vi "Dark Current Test with Manual Measurment.vi"() -> ()   [LabVIEW 2018]
uses:
  <vilib>/Utility/file.llb/Write Delimited Spreadsheet (string).vi
  <vilib>/Utility/file.llb/Write Delimited Spreadsheet (DBL).vi
  <instrlib>/CAEN PSM/CAEN PSM.lvlib
panel:
  out "Power Supply Trip":bool
  out "Time Left (s)":dbl
  out "8":bool
  out "7":bool
  out "6":bool
  out "5":bool
  out "4":bool
  out "3":bool
  out "2":bool
  out "1":bool
  out "Test is Running":bool
  in  "Begin Test":bool
  out "Manual Measurments \nNeeded":bool
  out "OVV? 2":bool=TRUE
  out "OVC? 2":bool=TRUE
  out "Actual Voltage Level (V) 2":dbl format="%#_13g"
  out "Recorded Current\nfor Previous Tube":dbl format="%#_13g"
  in  "Measure Next Tube":bool
  in  "Barcodes":string[](array[string])
  out "Next Measurment":string
  in  "N":i32
  in  "dt (s)":i32
  out "Actual Current Limit (nA)":dbl format="%#_13g"
  out "Actual Voltage Level (V)":dbl format="%#_13g"
  out "OVC?":bool=TRUE
  out "OVV?":bool=TRUE
  in  "Channel #":i32
  in  "VISA resource name":refnum<visa-resource-name>
  # "Dark Current Test"
  # "Instructions in Brief:\n1. Begin the program by clicking the white arrow.\n2. Assemble tubes into the test bench.\n3. Select COM5 for the \"VISA resource name\".\n4. Enter in how often you want to take measurement in the \"dt\" box (typically 60s)\n5. Enter in how many measurments you want to take (typically 15)\n6. Scan in the 8 tubes that you are testing.\n(If you take 15 measurments every 60s, the test will take 15 min.)\n7. Click \"Begin Test\". The \"Test is Running\" LED should light up.\n8. After the intial test, if the total current is below 16nA, \n    the program will write the \n     file and end the test.\n9. If the total current is above 16nA, manual\n    measurments need to be taken.\n10. Engage only the tube indicated by \"Next Measurment\". \n11. Click \"Measure\".\n12. Engage the next tube and continue untill all have been measured.\n13. In both cases, the program will write files and end the test. \n14. The test is over when the \"Test is Running\" LED has turned off."
  # "Green lights indicate tubes that have passed."
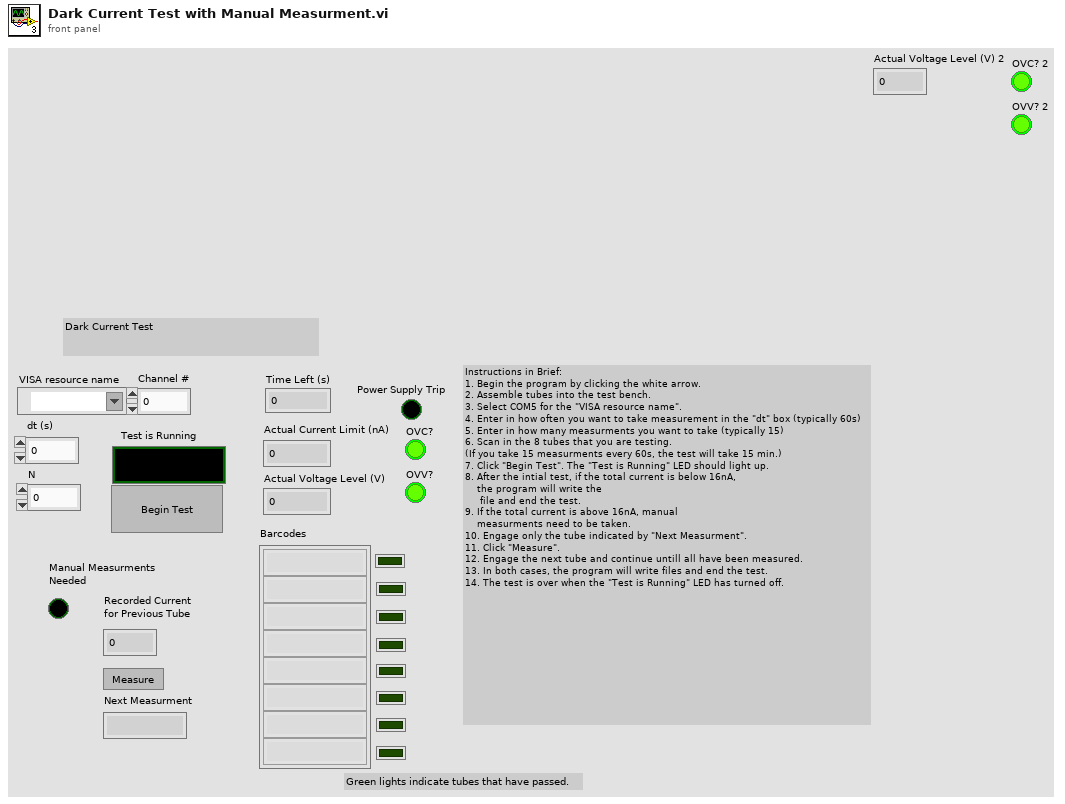
[diagram p1: front panel]
types:
  T1 = typedef "CAEN PSM.lvlib/BoardHandle.ctl" = cluster{"VISA resource name":refnum<visa-resource-name>, "Board address":u8, "NChannels":u8}
  T2 = cluster{"ON":bool, "RUP":bool, "RDW":bool, "OVC":bool, "OVV":bool, "UNV":bool, "MAXV":bool, "TRIP":bool, "OVP":bool, "OVT":bool, "DIS":bool, "KILL":bool, "ILK":bool, "NOCAL":bool}[]
  T3 = cluster{"ON":bool, "RUP":bool, "RDW":bool, "OVC":bool, "OVV":bool, "UNV":bool, "MAXV":bool, "TRIP":bool, "OVP":bool, "OVT":bool, "DIS":bool, "KILL":bool, "ILK":bool, "NOCAL":bool}
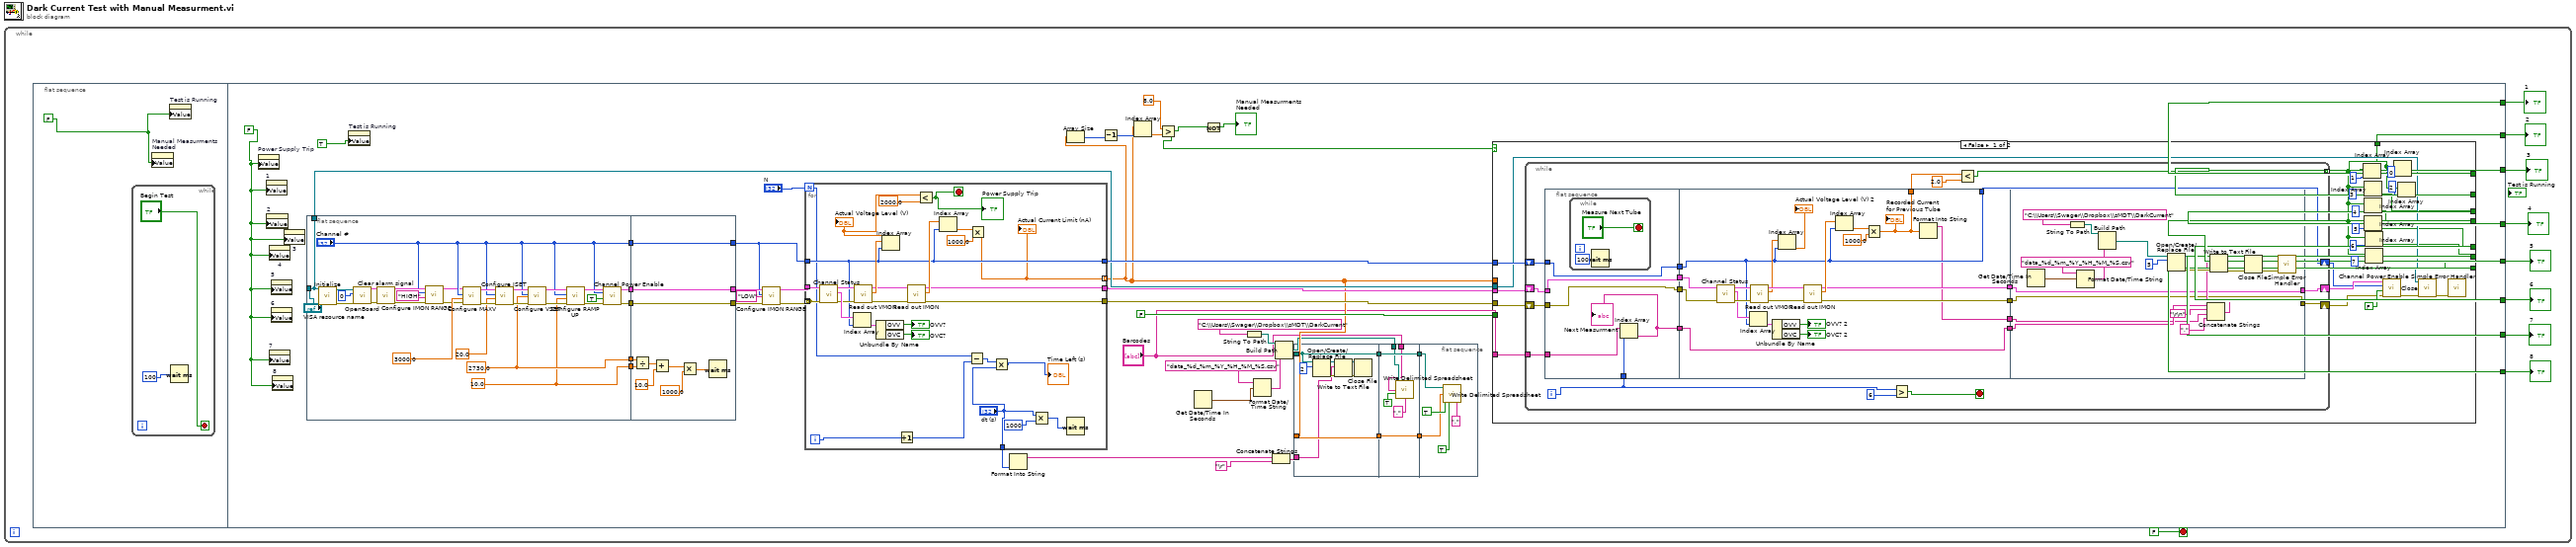
[diagram p0: block diagram]
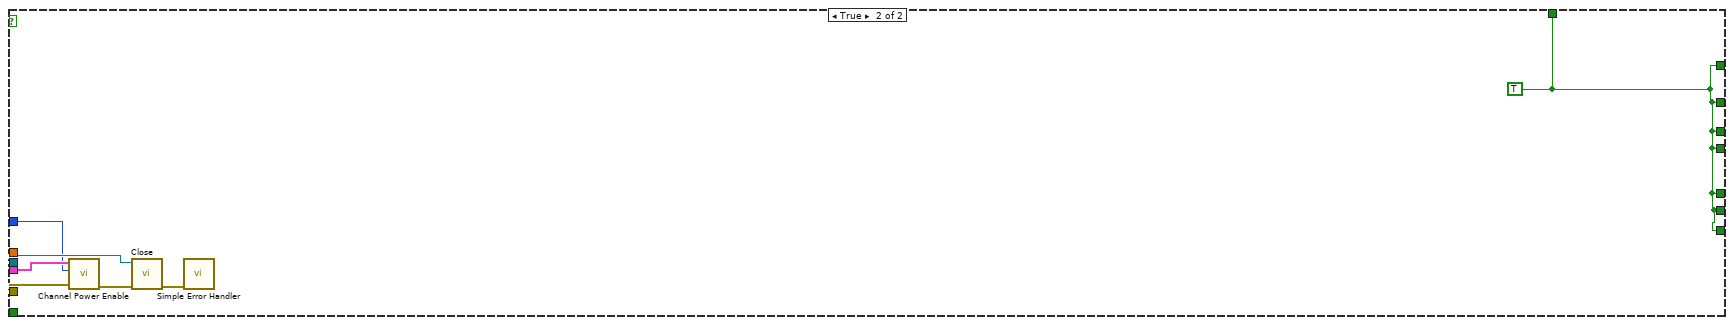
[diagram p2: hidden frame]
diagram:
  n1 = while {
    stop <- FALSE stop-if-true
    n2 = flat-sequence {
      tunnel: [w37] -> w8
      tunnel: [w36] -> w7
      tunnel: [w35] -> w6
      tunnel: [w34] -> w5
      tunnel: [w33] -> w4
      tunnel: [w32] -> w3
      tunnel: [w31] -> w2
      tunnel: [w30] -> w1
      frame #0 {
        w10 = FALSE
        n3 = while {
          stop <- "Begin Test" stop-if-true
          n4 = Wait (ms)(milliseconds to wait=100) -> ()  [unwired: 1 out]
        }
        n5 = property on="Manual Measurments \nNeeded" class="Bool (strict)"("Value"=w10) -> ()  [unwired: 2 in, 2 out]
        n6 = property on="Test is Running" class="Bool (strict)"("Value"=w10) -> ()  [unwired: 2 in, 2 out]
      }
      frame #1 {
        w23 = FALSE
        n7 = property on="Power Supply Trip" class="Bool (strict)"("Value"=w23) -> ()  [unwired: 2 in, 2 out]
        n8 = property on="1" class="Bool (strict)"("Value"=w23) -> ()  [unwired: 2 in, 2 out]
        n9 = property on="2" class="Bool (strict)"("Value"=w23) -> ()  [unwired: 2 in, 2 out]
        n10 = property on="4" class="Bool (strict)"("Value"=w23) -> ()  [unwired: 2 in, 2 out]
        n11 = property on="7" class="Bool (strict)"("Value"=w23) -> ()  [unwired: 2 in, 2 out]
        n12 = property on="5" class="Bool (strict)"("Value"=w23) -> ()  [unwired: 2 in, 2 out]
        n13 = property on="6" class="Bool (strict)"("Value"=w23) -> ()  [unwired: 2 in, 2 out]
        n14 = property on="8" class="Bool (strict)"("Value"=w23) -> ()  [unwired: 2 in, 2 out]
        n15 = property on="3" class="Bool (strict)"("Value"=w23) -> ()  [unwired: 2 in, 2 out]
        n16 = flat-sequence {
          tunnel: [w197] -> w62
          tunnel: [w196] -> w61
          tunnel: [w193] -> w52
          tunnel: [w195] -> w60
          tunnel: [w194] -> w59
          tunnel: ["Channel #"] -> w58
          tunnel: "VISA resource name" -> [w193]
          tunnel: w62 -> [w217]
          tunnel: w61 -> [w216]
          tunnel: [w215] -> w49
          tunnel: w60 -> [w215]
          tunnel: [w214] -> w50
          tunnel: w59 -> [w214]
          tunnel: [w213] -> w47
          tunnel: w58 -> [w213]
          frame #0 {
            w197 = 2730.0 ("Voltage Set (Volts)")
            w196 = 10.0 ("Voltage Ramp Up (V/s)")
            n17 = call <instrlib>:"Initialize.vi"("VISA resource name"=w193) -> ("error out"=w207:errorcluster, "VISA resource name out"=w203:refnum<visa-resource-name>)  [unwired: 9 in]
            n18 = call <instrlib>:"OpenBoard.vi"("error in (no error)"=w207, "Board Address"=0, "VISA resource name"=w203) -> ("error out"=w208:errorcluster, "BoardHandle"=w202:T1)  [unwired: 7 in]
            n19 = call <instrlib>:"Clear alarm signal.vi"("error in (no error)"=w208, "BoardHandle"=w202) -> ("error out"=w191:errorcluster, "BoardHandle out"=w190:T1)  [unwired: 8 in]
            n20 = call <instrlib>:"Configure IMON RANGE.vi"("error in (no error)"=w191, "IMon range (LOW)"="HIGH", "Channel (0)"="Channel #", "BoardHandle"=w190) -> ("error out"=w186:errorcluster, "BoardHandle out"=w187:T1)  [unwired: 6 in]
            n21 = call <instrlib>:"Configure MAXV.vi"("error in (no error)"=w186, "Voltage Max (0.0 V)"=3000.0 ("VMax (Volts)"), "Channel (0)"="Channel #", "BoardHandle"=w187) -> ("error out"=w209:errorcluster, "BoardHandle out"=w201:T1)  [unwired: 6 in]
            n22 = call <instrlib>:"Configure ISET.vi"("error in (no error)"=w209, "Current Limit (0.00 uA)"=20.0 ("Current Limit (uA)"), "Channel (0)"="Channel #", "BoardHandle"=w201) -> ("error out"=w210:errorcluster, "BoardHandle out"=w200:T1)  [unwired: 6 in]
            n23 = call <instrlib>:"Configure VSET.vi"("error in (no error)"=w210, "Voltage Level (0.0 V)"=w197, "Channel (0)"="Channel #", "BoardHandle"=w200) -> ("error out"=w211:errorcluster, "BoardHandle out"=w199:T1)  [unwired: 6 in]
            n24 = call <instrlib>:"Configure RAMP UP.vi"("error in (no error)"=w211, "Voltage ramp up (0 V/s)"=w196, "Channel (0)"="Channel #", "BoardHandle"=w199) -> ("error out"=w212:errorcluster, "BoardHandle out"=w198:T1)  [unwired: 6 in]
            n25 = call <instrlib>:"Channel Power Enable.vi"("error in (no error)"=w212, "Enable (OFF)"=TRUE ("Boolean"), "Channel (0)"="Channel #", "BoardHandle"=w198) -> ("error out"=w194:errorcluster, "BoardHandle out"=w195:T1)  [unwired: 6 in]
          }
          frame #1 {
            n26 = Divide(x=w217, y=w216) -> (x/y=w220:dbl)
            n27 = Add(x=w220, y=10.0) -> (x+y=w221:dbl)
            n28 = Multiply(x=w221, y=1000.0) -> (x*y=w222:dbl)
            n29 = Wait (ms)(milliseconds to wait=w222) -> ()  [unwired: 1 out]
          }
        }
        n30 = property on="Test is Running" class="Bool (strict)"("Value"=TRUE) -> ()  [unwired: 2 in, 2 out]
        n31 = call <instrlib>:"Configure IMON RANGE.vi"("error in (no error)"=w50, "IMon range (LOW)"="LOW", "Channel (0)"=w47, "BoardHandle"=w49) -> ("error out"=w45:errorcluster, "BoardHandle out"=w46:T1)  [unwired: 6 in]
        n32 = for {
          N: "N" -> [w231]
          tunnel: w45 -> [w238]
          tunnel: w47 -> [w239]
          tunnel: [w241] -> w56
          tunnel: [w240] -> w55
          tunnel: [w232] -> w24 mode=indexing
          tunnel: [w239] -> w53
          tunnel: w46 -> [w235]
          tunnel: [w238] -> _ mode=indexing
          tunnel: ["dt (s)"] -> w22
          i -> [w228]
          stop <- w226 stop-if-true
          n33 = call <instrlib>:"Channel Status.vi"("error in (no error)"=w238, "BoardHandle"=w235) -> ("error out"=w247:errorcluster, "Channel Status Array"=w251:T2, "BoardHandle out"=w246:T1)  [unwired: 7 in]
          n34 = Index Array(array=w251, index=w239) -> (element=w250:T3)
          n35 = call <instrlib>:"Read out VMON.vi"("error in (no error)"=w247, "BoardHandle"=w246) -> ("error out"=w243:errorcluster, "VMon values (V)"=w245:dbl[], "BoardHandle out"=w244:T1)  [unwired: 7 in]
          n36 = Unbundle By Name(w250) -> ("OVV"=→"OVV?":bool, "OVC"=→"OVC?":bool)
          n37 = Index Array(array=w245, index=w239) -> (element=w225:dbl)
          "Actual Voltage Level (V)" <- w225
          n38 = Increment(x=w228) -> (x+1=w227:i32)
          n39 = call <instrlib>:"Read out IMON.vi"("error in (no error)"=w243, "BoardHandle"=w244) -> ("error out"=w240:errorcluster, "IMon values (uA)"=w242:dbl[], "BoardHandle out"=w241:T1)  [unwired: 6 in, 1 out]
          n40 = Less?(x=w225, y=2000.0) -> (x < y?=w226:bool)
          "Power Supply Trip" <- w226
          n41 = Index Array(array=w242, index=w239) -> (element=w234:dbl)
          n42 = Subtract(x=w231, y=w227) -> (x-y=w230:i32)
          n43 = Multiply(x=w234, y=1000.0) -> (x*y=w232:dbl)
          "Actual Current Limit (nA)" <- w232
          n44 = Multiply(x=w230, y="dt (s)") -> (x*y=→"Time Left (s)":i32)
          n45 = Multiply(x="dt (s)", y=1000) -> (x*y=w237:i32)
          n46 = Wait (ms)(milliseconds to wait=w237) -> ()  [unwired: 1 out]
        }
        n47 = Format Into String(w22) -> (resulting string=w14:string)  [unwired: 3 in, 1 out]
        n48 = Array Size(array=w24) -> (size(s)=w44:i32)
        n49 = Decrement(x=w44) -> (x-1=w43:i32)
        n50 = Index Array(array=w24, index=w43) -> (element=w42:dbl)
        n51 = Greater?(x=8.0, y=w42) -> (0:w41:bool)
        n52 = Get Date/Time In Seconds() -> (seconds since 1Jan1904=w27:timestamp)
        n53 = Not(x=w41) -> (.not. x?=→"Manual Measurments \nNeeded":bool)
        n54 = String To Path(string="C:\\Users\\Swager\\Dropbox\\sMDT\\DarkCurrent") -> (path=w26:path)
        n55 = Format Date/Time String(time format string (%c)="data_%d_%m_%Y_%H_%M_%S.csv", seconds (now)=w27) -> (date/time string=w28:string)  [unwired: 1 in]
        n56 = Concatenate Strings(w14, "\r") -> (w15:string)
        n57 = Build Path(base path=w26, name or relative path=w28) -> (appended path=w17:path)
        n58 = flat-sequence {
          tunnel: w17 -> [w69]
          tunnel: [w69] -> w21
          tunnel: [w70] -> w19
          tunnel: w24 -> [w70]
          tunnel: w15 -> [w66]
          tunnel: w21 -> [w76]
          tunnel: [w76] -> w20
          tunnel: w19 -> [w75]
          tunnel: [w75] -> w18
          tunnel: w17 -> [w74]
          tunnel: "Barcodes" -> [w73]
          tunnel: w20 -> [w79]
          tunnel: w18 -> [w78]
          frame #0 {
            n59 = Open/Create/Replace File(file path (use dialog)=w69, operation (0:open)=2) -> (refnum out=w67:refnum<file>, error out=w68:errorcluster)  [unwired: 4 in, 1 out]
            n60 = Write to Text File(file (use dialog)=w67, text=w66, error in=w68) -> (refnum out=w64:refnum<file>, error out=w65:errorcluster)  [unwired: 1 in, 1 out]
            n61 = Close File(refnum=w64, error in=w65) -> ()  [unwired: 2 out]
          }
          frame #1 {
            n62 = call-poly <vilib>:"Write Delimited Spreadsheet.vi"("file path (dialog if empty)"=w74, "1D data"=w73, "append to file? (new file:F)"=TRUE, "delimiter (\\t)"=",") -> ()  [unwired: 10 in, 2 out]
          }
          frame #2 {
            n63 = call-poly <vilib>:"Write Delimited Spreadsheet.vi"("file path (dialog if empty)"=w79, "1D data"=w78, "append to file? (new file:F)"=TRUE, "transpose? (no:F)"=TRUE, "delimiter (\\t)"=",") -> ()  [unwired: 9 in, 2 out]
          }
        }
        n64 = case shown="False" w41 {
          tunnel: w56 -> [w108 w181]
          tunnel: w55 -> [w109 w180]
          tunnel: FALSE -> [_ _]
          tunnel: w53 -> [w107 w179]
          tunnel: w52 -> [w103 w182]
          tunnel: w24 -> [_ _]
          tunnel: "Barcodes" -> [w99 _]
          tunnel: [w89 w185] -> w37
          tunnel: [w88 w185] -> w36
          tunnel: [w87 w185] -> w35
          tunnel: [w86 w185] -> w34
          tunnel: [w85 w185] -> w33
          tunnel: [w84 w185] -> w32
          tunnel: [w83 w185] -> w31
          tunnel: [w82 w185] -> w30
          frame False {
            n65 = while {
              shift-right: [w115] -> w100
              shift-left: w107 -> [w125]
              shift-right: [w117] -> w102
              shift-left: w108 -> [w122]
              shift-right: [w116] -> w101
              shift-left: w109 -> [w120]
              tunnel: w99 -> [w113]
              tunnel: [w110] -> w98 mode=indexing
              i -> [w128]
              stop <- w129 stop-if-true
              n66 = flat-sequence {
                tunnel: w128 -> [w136]
                tunnel: [w135] -> w127
                tunnel: w125 -> [w134]
                tunnel: [w134] -> w124
                tunnel: [w133] -> w123
                tunnel: w122 -> [w133]
                tunnel: [w132] -> w121
                tunnel: w120 -> [w132]
                tunnel: w113 -> [w131]
                tunnel: w127 -> [w146]
                tunnel: [w146] -> w126
                tunnel: w124 -> [w141]
                tunnel: w123 -> [w144]
                tunnel: w121 -> [w145]
                tunnel: [w143] -> w119
                tunnel: [w142] -> w118
                tunnel: [w141] -> w115
                tunnel: [w140] -> w114
                tunnel: [w139] -> w112
                tunnel: w126 -> [w164]
                tunnel: w119 -> [w162]
                tunnel: w118 -> [w161]
                tunnel: [w162] -> w117
                tunnel: [w161] -> w116
                tunnel: w114 -> [w160]
                frame #0 {
                  n67 = while {
                    stop <- "Measure Next Tube" stop-if-true
                    n68 = Wait (ms)(milliseconds to wait=100) -> ()  [unwired: 1 out]
                  }
                  n69 = Index Array(array=w131, index=w136) -> (element=w135:string)
                  "Next Measurment" <- w135
                }
                frame #1 {
                  n70 = call <instrlib>:"Channel Status.vi"("error in (no error)"=w145, "BoardHandle"=w144) -> ("error out"=w152:errorcluster, "Channel Status Array"=w148:T2, "BoardHandle out"=w153:T1)  [unwired: 7 in]
                  n71 = Index Array(array=w148, index=w141) -> (element=w149:T3)
                  n72 = call <instrlib>:"Read out VMON.vi"("error in (no error)"=w152, "BoardHandle"=w153) -> ("error out"=w156:errorcluster, "VMon values (V)"=w154:dbl[], "BoardHandle out"=w155:T1)  [unwired: 7 in]
                  n73 = Unbundle By Name(w149) -> ("OVV"=→"OVV? 2":bool, "OVC"=→"OVC? 2":bool)
                  n74 = Index Array(array=w154, index=w141) -> (element=→"Actual Voltage Level (V) 2":dbl)
                  n75 = call <instrlib>:"Read out IMON.vi"("error in (no error)"=w156, "BoardHandle"=w155) -> ("error out"=w142:errorcluster, "IMon values (uA)"=w159:dbl[], "BoardHandle out"=w143:T1)  [unwired: 6 in, 1 out]
                  n76 = Index Array(array=w159, index=w141) -> (element=w157:dbl)
                  n77 = Multiply(x=w157, y=1000.0) -> (x*y=w139:dbl)
                  "Recorded Current\nfor Previous Tube" <- w139
                  n78 = Format Into String(w139) -> (resulting string=w140:string)  [unwired: 3 in, 1 out]
                }
                frame #2 {
                  n79 = Get Date/Time In Seconds() -> (seconds since 1Jan1904=w176:timestamp)
                  n80 = String To Path(string="C:\\Users\\Swager\\Dropbox\\sMDT\\DarkCurrent") -> (path=w175:path)
                  n81 = Format Date/Time String(time format string (%c)="data_%d_%m_%Y_%H_%M_%S.csv", seconds (now)=w176) -> (date/time string=w177:string)  [unwired: 1 in]
                  n82 = Build Path(base path=w175, name or relative path=w177) -> (appended path=w173:path)
                  n83 = Open/Create/Replace File(file path (use dialog)=w173, operation (0:open)=5) -> (refnum out=w172:refnum<file>, error out=w171:errorcluster)  [unwired: 4 in, 1 out]
                  n84 = Concatenate Strings(w164, "\r\n", w160, ",") -> (w166:string)
                  n85 = Write to Text File(file (use dialog)=w172, text=w166, error in=w171) -> (refnum out=w170:refnum<file>, error out=w169:errorcluster)  [unwired: 1 in, 1 out]
                  n86 = Close File(refnum=w170, error in=w169) -> (error out=w168:errorcluster)  [unwired: 1 out]
                  n87 = call <vilib>:"Simple Error Handler.vi"("error in (no error)"=w168) -> ()  [unwired: 4 in, 5 out]
                }
              }
              n88 = Greater?(x=w128, y=6) -> (0:w129:bool)
              n89 = Less?(x=w112, y=2.0) -> (x < y?=w110:bool)
            }
            n90 = Index Array(array=w98, index=1) -> (element=w88:bool)
            n91 = Index Array(array=w98, index=3) -> (element=w86:bool)
            n92 = Index Array(array=w98, index=4) -> (element=w85:bool)
            n93 = Index Array(array=w98, index=5) -> (element=w84:bool)
            n94 = Index Array(array=w98, index=6) -> (element=w83:bool)
            n95 = Index Array(array=w98, index=7) -> (element=w82:bool)
            n96 = call <instrlib>:"Channel Power Enable.vi"("error in (no error)"=w101, "Enable (OFF)"=FALSE, "Channel (0)"=w100, "BoardHandle"=w102) -> ("error out"=w105:errorcluster)  [unwired: 6 in, 1 out]
            n97 = Index Array(array=w98, index=0) -> (element=w89:bool)
            n98 = Index Array(array=w98, index=2) -> (element=w87:bool)
            n99 = call <instrlib>:"Close.vi"("error in (no error)"=w105, "VISA resource name"=w103) -> ("error out"=w104:errorcluster)  [unwired: 9 in]
            n100 = call <vilib>:"Simple Error Handler.vi"("error in (no error)"=w104) -> ()  [unwired: 4 in, 5 out]
          }
          frame True {
            w185 = TRUE
            n101 = call <instrlib>:"Channel Power Enable.vi"("error in (no error)"=w180, "Channel (0)"=w179, "BoardHandle"=w181) -> ("error out"=w184:errorcluster)  [unwired: 7 in, 1 out]
            n102 = call <instrlib>:"Close.vi"("error in (no error)"=w184, "VISA resource name"=w182) -> ("error out"=w183:errorcluster)  [unwired: 9 in]
            n103 = call <vilib>:"Simple Error Handler.vi"("error in (no error)"=w183) -> ()  [unwired: 4 in, 5 out]
          }
        }
      }
    }
    "1" <- w8
    "2" <- w7
    "3" <- w6
    "4" <- w5
    "5" <- w4
    "8" <- w1
    "6" <- w3
    "7" <- w2
  }
